vi "GetHardwareInfo.vi"(7 "LabVIEW Web Service Request":refnum<class "Web Request.lvclass">) -> ()   [LabVIEW 2015]
uses:
  <vilib>/wsapi/Web Request.lvclass
  <vilib>/addons/SystemInfoProcess/SystemInfoProcess.lvlib
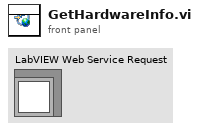
[diagram p1: front panel]
types:
  T1 = typedef "cRIODetectHW.lvlib/SystemHW.ctl" = cluster{"controller":T2, "chassis":T2, "modules":T2[]}
  T2 = typedef "cRIODetectHW.lvlib/cRIO Product Info.ctl" = cluster{"vendorName":string, "productName":string, "serialNumber":string}
  T3 = typedef "KeyValuePair.ctl" = cluster{"Key":string, "Value":string}
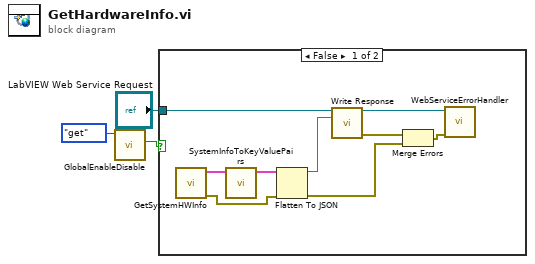
[diagram p0: block diagram]
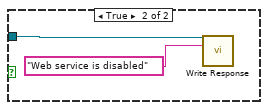
[diagram p2: hidden frame]
diagram:
  n1 = call "GlobalEnableDisable.vi"("action"=enum16{"init", "set", "get"}."get") -> ("DisableDeviceWebService"=w1:bool)  [unwired: 10 in]
  n2 = case shown="False" w1 {
    tunnel: "LabVIEW Web Service Request" -> [w12 w13]
    frame False {
      n3 = call <vilib>:"GetSystemHWInfo.vi"() -> ("error out"=w5:errorcluster, "system info"=w8:T1)  [unwired: 9 in, 1 out]
      n4 = call "SystemInfoToKeyValuePairs.vi"("system info"=w8) -> ("hardware info key value pair"=w7:T3[])  [unwired: 10 in]
      n5 = Flatten To JSON(anything=w7, error in (no error)=w5) -> (JSON string=w11:string, 11:w4:errorcluster)  [unwired: 1 in]
      n6 = call <vilib>:"Write Response.vi"("LabVIEW Web Service Request"=w12, "response string"=w11) -> ("LabVIEW Web Service Request out"=w10:refnum<class "Web Request.lvclass">, "error out"=w9:errorcluster)  [unwired: 12 in]
      n7 = Merge Errors(w9, w4) -> (w6:errorcluster)
      n8 = call "WebServiceErrorHandler.vi"("LabVIEW Web Service Request"=w10, "error in (no error)"=w6) -> ()  [unwired: 12 in, 2 out]
    }
    frame True {
      n9 = call <vilib>:"Write Response.vi"("LabVIEW Web Service Request"=w13, "response string"="Web service is disabled") -> ()  [unwired: 12 in, 2 out]
    }
  }
